vi "LogonUser.vi"() -> ()   [LabVIEW 2018]
doc: "©2019\nWiebe Walstra\nwww.carya.nl"
uses:
  kernel32.dll
  advapi32.dll
panel:
  out "Name before":string
  out "success 4":i32
  out "success 3":i32
  out "success 2":i32
  out "error out":errorcluster
  out "Name during":string
  out "Name after":string
  out "error":i32
  out "success":i32
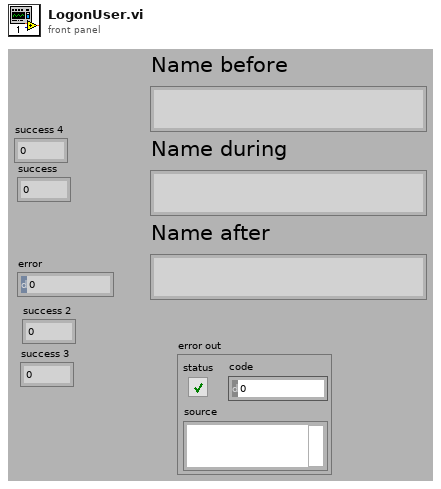
[diagram p1: front panel]
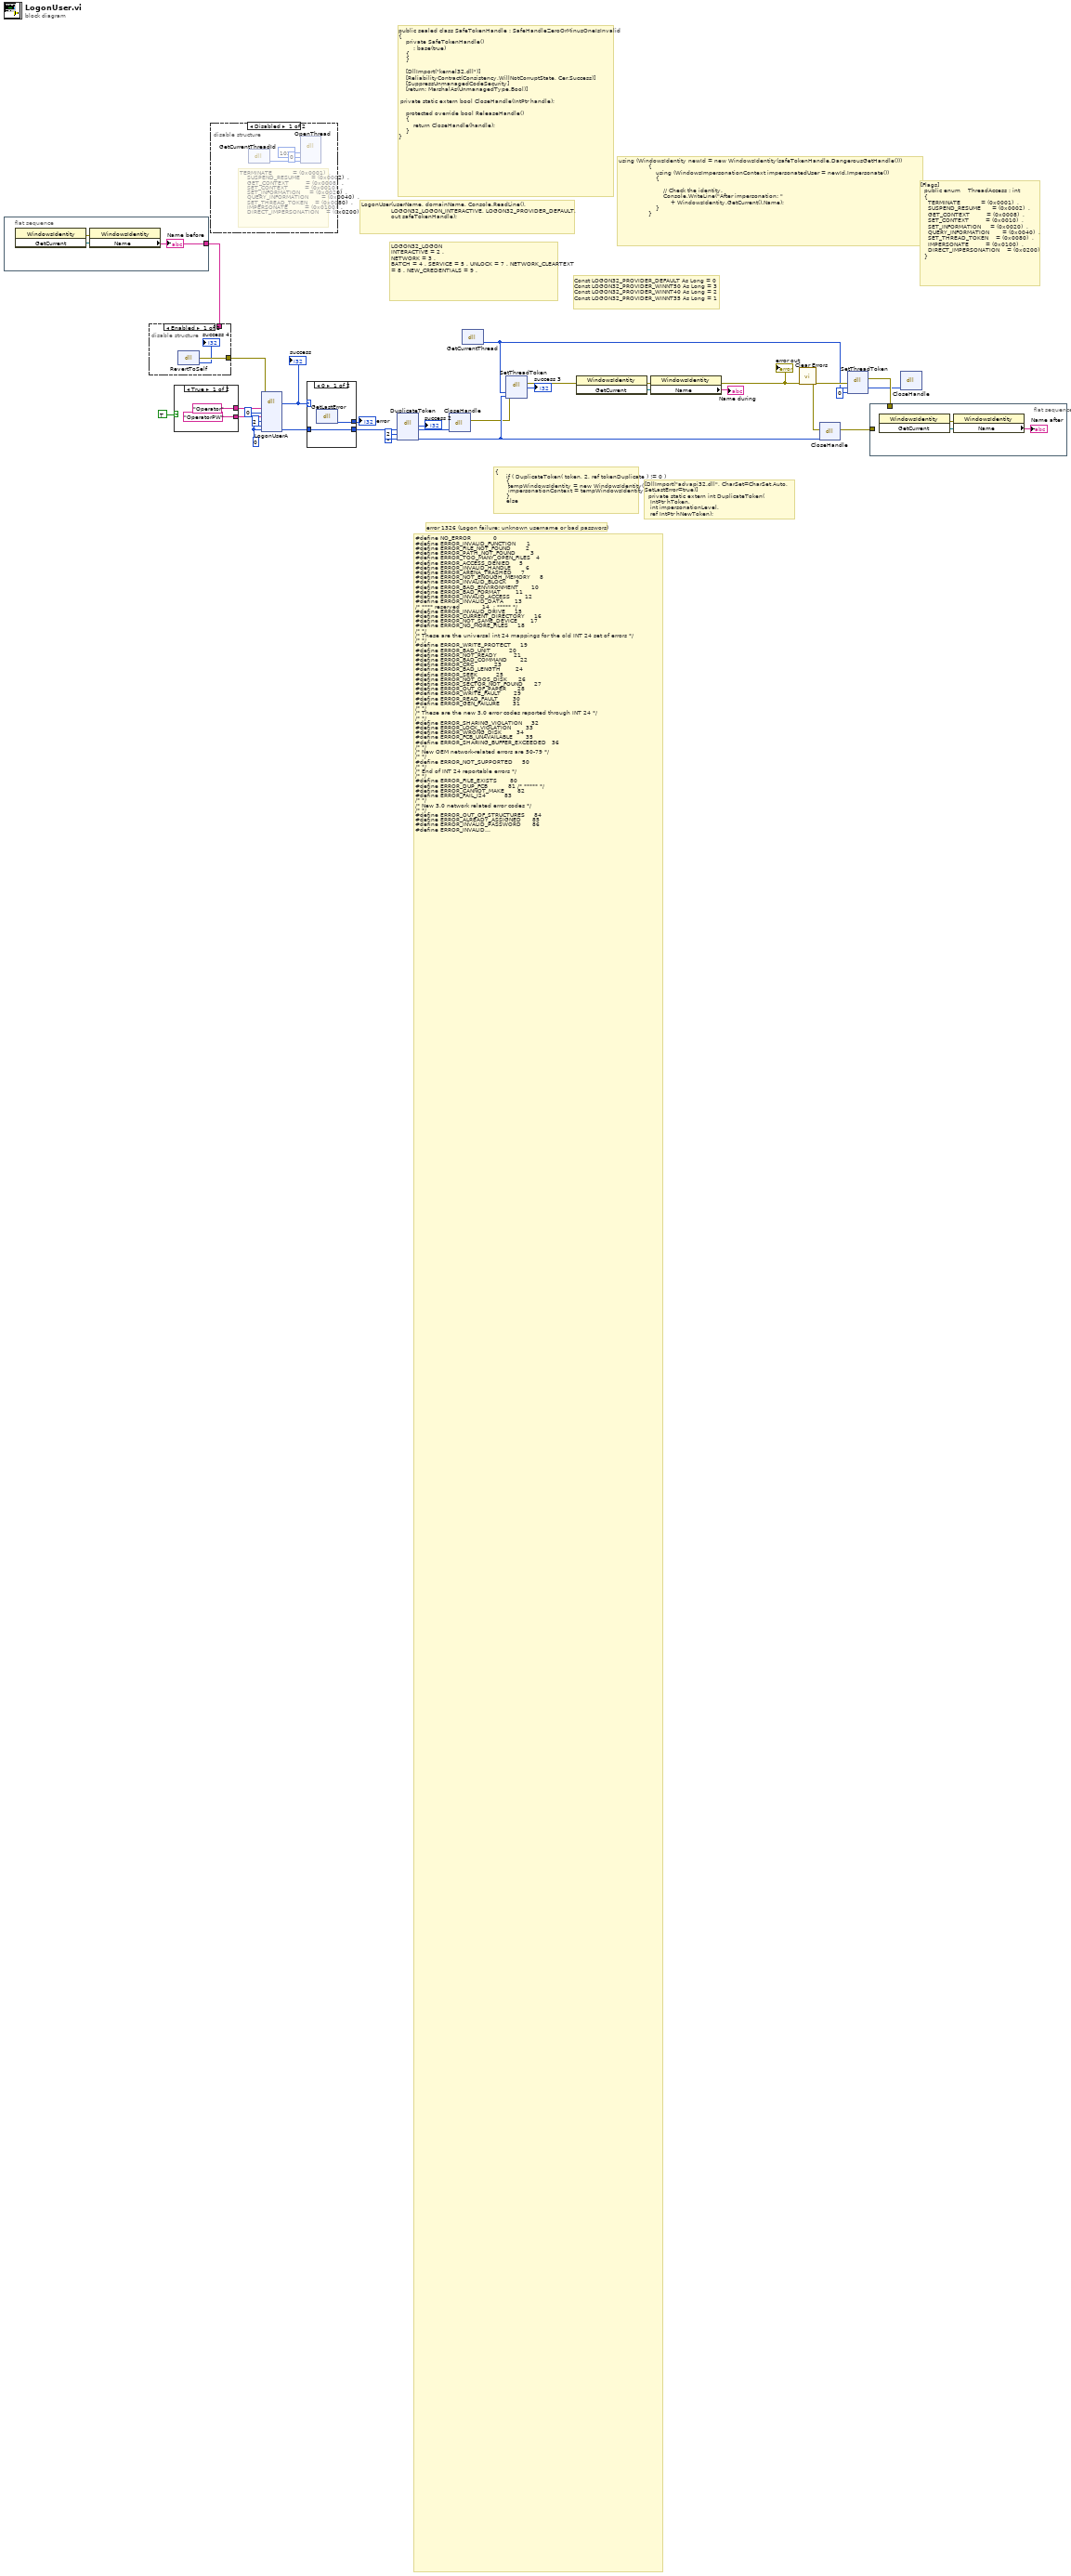
[diagram p0: block diagram]
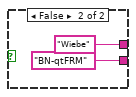
[diagram p5: hidden frame]
diagram:
  w27 = 0 ("dwLogonType")
  # "[Flags]\n  public enum    ThreadAccess : int\n  {\n    TERMINATE           = (0x0001)  ,\n    SUSPEND_RESUME      = (0x0002)  ,\n    GET_CONTEXT         = (0x0008)  ,\n    SET_CONTEXT         = (0x0010)  ,\n    SET_INFORMATION     = (0x0020)  ,\n    QUERY_INFORMATION       = (0x0040)  ,\n    SET_THREAD_TOKEN    = (0x0080)  ,\n    IMPERSONATE         = (0x0100)  ,\n    DIRECT_IMPERSONATION    = (0x0200)\n  }"
  # "[DllImport(\"advapi32.dll\", CharSet=CharSet.Auto, SetLastError=true)]\n\t\tprivate static extern int DuplicateToken(\n\t\t\tIntPtr hToken,\n\t\t\tint impersonationLevel,\n\t\t\tref IntPtr hNewToken);"
  # "{\n\t\t\t\t\t\tif ( DuplicateToken( token, 2, ref tokenDuplicate ) != 0 )\n\t\t\t\t\t\t{\n\t\t\t\t\t\t\ttempWindowsIdentity = new WindowsIdentity( tokenDuplicate );\n\t\t\t\t\t\t\timpersonationContext = tempWindowsIdentity.Impersonate();\n\t\t\t\t\t\t}\n\t\t\t\t\t\telse"
  # "public sealed class SafeTokenHandle : SafeHandleZeroOrMinusOneIsInvalid\n{\n    private SafeTokenHandle()\n        : base(true)\n    {\n    }\n\n    [DllImport(\"kernel32.dll\")]\n    [ReliabilityContract(Consistency.WillNotCorruptState, Cer.Success)]\n    [SuppressUnmanagedCodeSecurity]\n    [return: MarshalAs(UnmanagedType.Bool)]\n  \n private static extern bool CloseHandle(IntPtr handle);\n\n    protected override bool ReleaseHandle()\n    {\n        return CloseHandle(handle);\n    }\n}"
  # "LogonUser(userName, domainName, Console.ReadLine(),\n                LOGON32_LOGON_INTERACTIVE, LOGON32_PROVIDER_DEFAULT,\n                out safeTokenHandle);"
  # "using (WindowsIdentity newId = new WindowsIdentity(safeTokenHandle.DangerousGetHandle()))\n                {\n                    using (WindowsImpersonationContext impersonatedUser = newId.Impersonate())\n                    {\n\n                        // Check the identity.\n                        Console.WriteLine(\"After impersonation: \"\n                            + WindowsIdentity.GetCurrent().Name);\n                    }\n                }"
  # "Const LOGON32_PROVIDER_DEFAULT As Long = 0\nConst LOGON32_PROVIDER_WINNT50 As Long = 3\nConst LOGON32_PROVIDER_WINNT40 As Long = 2\nConst LOGON32_PROVIDER_WINNT35 As Long = 1"
  # "error 1326 (Logon failure: unknown username or bad passwors)"
  # "LOGON32_LOGON \nINTERACTIVE = 2 .\nNETWORK = 3 .\nBATCH = 4 . SERVICE = 5 . UNLOCK = 7 . NETWORK_CLEARTEXT = 8 . NEW_CREDENTIALS = 9 ."
  # "#define NO_ERROR            0\n#define ERROR_INVALID_FUNCTION      1\n#define ERROR_FILE_NOT_FOUND        2\n#define ERROR_PATH_NOT_FOUND        3\n#define ERROR_TOO_MANY_OPEN_FILES   4\n#define ERROR_ACCESS_DENIED     5\n#define ERROR_INVALID_HANDLE        6\n#define ERROR_ARENA_TRASHED     7\n#define ERROR_NOT_ENOUGH_MEMORY     8\n#define ERROR_INVALID_BLOCK     9\n#define ERROR_BAD_ENVIRONMENT       10\n#define ERROR_BAD_FORMAT        11\n#define ERROR_INVALID_ACCESS        12\n#define ERROR_INVALID_DATA      13\n/* **** reserved            14  ; ***** */\n#define ERROR_INVALID_DRIVE     15\n#define ERROR_CURRENT_DIRECTORY     16\n#define ERROR_NOT_SAME_DEVICE       17\n#define ERROR_NO_MORE_FILES     18\n/* */\n/* These are the universal int 24 mappings for the old INT 24 set of errors */\n/* */\n#define ERROR_WRITE_PROTECT     19\n#define ERROR_BAD_UNIT          20\n#define ERROR_NOT_READY         21\n#define ERROR_BAD_COMMAND       22\n#define ERROR_CRC           23\n#define ERROR_BAD_LENGTH        24\n#define ERROR_SEEK          25\n#define ERROR_NOT_DOS_DISK      26\n#define ERROR_SECTOR_NOT_FOUND      27\n#define ERROR_OUT_OF_PAPER      28\n#define ERROR_WRITE_FAULT       29\n#define ERROR_READ_FAULT        30\n#define ERROR_GEN_FAILURE       31\n/* */\n/* These are the new 3.0 error codes reported through INT 24 */\n/* */\n#define ERROR_SHARING_VIOLATION     32\n#define ERROR_LOCK_VIOLATION        33\n#define ERROR_WRONG_DISK        34\n#define ERROR_FCB_UNAVAILABLE       35\n#define ERROR_SHARING_BUFFER_EXCEEDED   36\n/* */\n/* New OEM network-related errors are 50-79 */\n/* */\n#define ERROR_NOT_SUPPORTED     50\n/* */\n/* End of INT 24 reportable errors */\n/* */\n#define ERROR_FILE_EXISTS       80\n#define ERROR_DUP_FCB           81 /* ***** */\n#define ERROR_CANNOT_MAKE       82\n#define ERROR_FAIL_I24          83\n/* */\n/* New 3.0 network related error codes */\n/* */\n#define ERROR_OUT_OF_STRUCTURES     84\n#define ERROR_ALREADY_ASSIGNED      85\n#define ERROR_INVALID_PASSWORD      86\n#define ERROR_INVALID_PARAMETER     87\n#define ERROR_NET_WRITE_FAULT       88\n/* */\n/* New error codes for 4.0 */\n/* */\n#define ERROR_NO_PROC_SLOTS     89  /* no process slots available */\n#define ERROR_NOT_FROZEN        90\n#define ERR_TSTOVFL         91  /* timer service table overflow */\n#define ERR_TSTDUP          92  /* timer service table duplicate */\n#define ERROR_NO_ITEMS          93  /* There were no items to operate upon */\n#define ERROR_INTERRUPT         95  /* interrupted system call */\n\n#define ERROR_TOO_MANY_SEMAPHORES   100\n#define ERROR_EXCL_SEM_ALREADY_OWNED    101\n#define ERROR_SEM_IS_SET        102\n#define ERROR_TOO_MANY_SEM_REQUESTS 103\n#define ERROR_INVALID_AT_INTERRUPT_TIME 104\n\n#define ERROR_SEM_OWNER_DIED        105 /* waitsem found owner died */\n#define ERROR_SEM_USER_LIMIT        106 /* too many procs have this sem */\n#define ERROR_DISK_CHANGE       107 /* insert disk b into drive a */\n#define ERROR_DRIVE_LOCKED      108 /* drive locked by another process */\n#define ERROR_BROKEN_PIPE       109 /* write on pipe with no reader */\n/* */\n/* New error codes for OS/2 */\n/* */\n#define ERROR_OPEN_FAILED       110 /* open/created failed due to */\n                        /* explicit fail command */\n#define ERROR_BUFFER_OVERFLOW       111 /* buffer passed to system call */\n                        /* is too small to hold return */\n                        /* data. */\n#define ERROR_DISK_FULL         112 /* not enough space on the disk */\n                        /* (DOSNEWSIZE/w_NewSize) */\n#define ERROR_NO_MORE_SEARCH_HANDLES    113 /* can't allocate another search */\n                        /* structure and handle. */\n                        /* (DOSFINDFIRST/w_FindFirst) */\n#define ERROR_INVALID_TARGET_HANDLE 114 /* Target handle in DOSDUPHANDLE */\n                        /* is invalid */\n#define ERROR_PROTECTION_VIOLATION  115 /* Bad user virtual address */\n#define ERROR_VIOKBD_REQUEST        116\n#define ERROR_INVALID_CATEGORY      117 /* Category for DEVIOCTL in not */\n                        /* defined */\n#define ERROR_INVALID_VERIFY_SWITCH 118 /* invalid value passed for */\n                        /* verify flag */\n#define ERROR_BAD_DRIVER_LEVEL      119 /* DosDevIOCTL looks for a level */\n                        /* four driver.   If the driver */\n                        /* is not level four we return */\n                        /* this code */\n#define ERROR_CALL_NOT_IMPLEMENTED  120 /* returned from stub api calls. */\n                        /* This call will disappear when */\n                        /* all the api's are implemented. */\n#define ERROR_SEM_TIMEOUT       121 /* Time out happened from the */\n                        /* semaphore api functions. */\n#define ERROR_INSUFFICIENT_BUFFER   122 /* Some call require the  */\n                        /* application to pass in a buffer */\n                        /* filled with data.  This error is */\n                        /* returned if the data buffer is too */\n                        /* small.  For example: DosSetFileInfo */\n                        /* requires 4 bytes of data.  If a */\n                        /* two byte buffer is passed in then */\n                        /* this error is returned.   */\n                        /* error_buffer_overflow is used when */\n                        /* the output buffer in not big enough. */\n#define ERROR_INVALID_NAME      123 /* illegal character or malformed */\n                        /* file system name */\n#define ERROR_INVALID_LEVEL     124 /* unimplemented level for info */\n                        /* retrieval or setting */\n#define ERROR_NO_VOLUME_LABEL       125 /* no volume label found with */\n                        /* DosQFSInfo command */\n#define ERROR_MOD_NOT_FOUND     126 /* w_getprocaddr,w_getmodhandle */\n#define ERROR_PROC_NOT_FOUND        127 /* w_getprocaddr */\n\n#define ERROR_WAIT_NO_CHILDREN      128 /* CWait finds to children */\n\n#define ERROR_CHILD_NOT_COMPLETE    129 /* CWait children not dead yet */\n\n/*This is a temporary fix for the 4-19-86 build this should be changed when */\n/* we get the file from MS */\n#define ERROR_DIRECT_ACCESS_HANDLE  130 /* handle operation is invalid */\n                        /* for direct disk access */\n                        /* handles */\n#define ERROR_NEGATIVE_SEEK     131 /* application tried to seek  */\n                        /* with negative offset */\n#define ERROR_SEEK_ON_DEVICE        132 /* application tried to seek */\n                        /* on device or pipe */\n/* */\n/* The following are errors generated by the join and subst workers */\n/* */\n#define ERROR_IS_JOIN_TARGET        133\n#define ERROR_IS_JOINED         134\n#define ERROR_IS_SUBSTED        135\n#define ERROR_NOT_JOINED        136\n#define ERROR_NOT_SUBSTED       137\n#define ERROR_JOIN_TO_JOIN      138\n#define ERROR_SUBST_TO_SUBST        139\n#define ERROR_JOIN_TO_SUBST     140\n#define ERROR_SUBST_TO_JOIN     141\n#define ERROR_BUSY_DRIVE        142\n#define ERROR_SAME_DRIVE        143\n#define ERROR_DIR_NOT_ROOT      144\n#define ERROR_DIR_NOT_EMPTY     145\n#define ERROR_IS_SUBST_PATH     146\n#define ERROR_IS_JOIN_PATH      147\n#define ERROR_PATH_BUSY         148\n#define ERROR_IS_SUBST_TARGET       149\n#define ERROR_SYSTEM_TRACE      150 /* system trace error */\n#define ERROR_INVALID_EVENT_COUNT   151 /* DosMuxSemWait errors */\n#define ERROR_TOO_MANY_MUXWAITERS   152\n#define ERROR_INVALID_LIST_FORMAT   153\n#define ERROR_LABEL_TOO_LONG        154\n#define ERROR_TOO_MANY_TCBS     155\n#define ERROR_SIGNAL_REFUSED        156\n#define ERROR_DISCARDED         157\n#define ERROR_NOT_LOCKED        158\n#define ERROR_BAD_THREADID_ADDR     159\n#define ERROR_BAD_ARGUMENTS     160\n#define ERROR_BAD_PATHNAME      161\n#define ERROR_SIGNAL_PENDING        162\n#define ERROR_UNCERTAIN_MEDIA       163\n#define ERROR_MAX_THRDS_REACHED     164\n#define ERROR_MONITORS_NOT_SUPPORTED    165\n\n#define ERROR_INVALID_SEGMENT_NUMBER    180\n#define ERROR_INVALID_CALLGATE      181\n#define ERROR_INVALID_ORDINAL       182\n#define ERROR_ALREADY_EXISTS        183\n#define ERROR_NO_CHILD_PROCESS      184\n#define ERROR_CHILD_ALIVE_NOWAIT    185\n#define ERROR_INVALID_FLAG_NUMBER   186\n#define ERROR_SEM_NOT_FOUND     187\n\n/*  following error codes have added to make the loader error\n    messages distinct\n*/\n\n#define ERROR_INVALID_STARTING_CODESEG  188\n#define ERROR_INVALID_STACKSEG      189\n#define ERROR_INVALID_MODULETYPE    190\n#define ERROR_INVALID_EXE_SIGNATURE 191\n#define ERROR_EXE_MARKED_INVALID    192\n#define ERROR_BAD_EXE_FORMAT        193\n#define ERROR_ITERATED_DATA_EXCEEDS_64k 194\n#define ERROR_INVALID_MINALLOCSIZE  195\n#define ERROR_DYNLINK_FROM_INVALID_RING 196\n#define ERROR_IOPL_NOT_ENABLED      197\n#define ERROR_INVALID_SEGDPL        198\n#define ERROR_AUTODATASEG_EXCEEDS_64k   199\n#define ERROR_RING2SEG_MUST_BE_MOVABLE  200\n#define ERROR_RELOC_CHAIN_XEEDS_SEGLIM  201\n#define ERROR_INFLOOP_IN_RELOC_CHAIN    202\n\n#define ERROR_ENVVAR_NOT_FOUND      203\n#define ERROR_NOT_CURRENT_CTRY      204\n#define ERROR_NO_SIGNAL_SENT        205\n#define ERROR_FILENAME_EXCED_RANGE  206 /* if filename > 8.3 */\n#define ERROR_RING2_STACK_IN_USE    207 /* for FAPI */\n#define ERROR_META_EXPANSION_TOO_LONG   208 /* if \"*a\" > 8.3 */\n\n#define ERROR_INVALID_SIGNAL_NUMBER 209\n#define ERROR_THREAD_1_INACTIVE     210\n#define ERROR_INFO_NOT_AVAIL        211 /*@@ PTM 5550 */\n#define ERROR_LOCKED            212\n#define ERROR_BAD_DYNALINK      213 /*@@ PTM 5760 */\n#define ERROR_TOO_MANY_MODULES      214\n#define ERROR_NESTING_NOT_ALLOWED   215\n\n/*\n * Error codes 230 - 249 are reserved for MS Networks\n */\n\n#define ERROR_USER_DEFINED_BASE     0xF000\n\n#define ERROR_I24_WRITE_PROTECT     0\n#define ERROR_I24_BAD_UNIT      1\n#define ERROR_I24_NOT_READY     2\n#define ERROR_I24_BAD_COMMAND       3\n#define ERROR_I24_CRC           4\n#define ERROR_I24_BAD_LENGTH        5\n#define ERROR_I24_SEEK          6\n#define ERROR_I24_NOT_DOS_DISK      7\n#define ERROR_I24_SECTOR_NOT_FOUND  8\n#define ERROR_I24_OUT_OF_PAPER      9\n#define ERROR_I24_WRITE_FAULT       0x0A\n#define ERROR_I24_READ_FAULT        0x0B\n#define ERROR_I24_GEN_FAILURE       0x0C\n#define ERROR_I24_DISK_CHANGE       0x0D\n#define ERROR_I24_WRONG_DISK        0x0F\n#define ERROR_I24_UNCERTAIN_MEDIA   0x10\n#define ERROR_I24_CHAR_CALL_INTERRUPTED 0x11\n#define ERROR_I24_NO_MONITOR_SUPPORT    0x12\n#define ERROR_I24_INVALID_PARAMETER 0x13"
  n1 = flat-sequence {
    tunnel: [w31] -> w13
    frame #0 {
      n2 = invoke class="WindowsIdentity" method="GetCurrent"() -> (error out=w32:errorcluster, "GetCurrent"=w33:refnum<k24>)  [unwired: 3 in, 1 out]
      n3 = property class="WindowsIdentity"(reference=w33, error in=w32) -> ("Name"=w31:string)  [unwired: 2 out]
      "Name before" <- w31
    }
  }
  n4 = disable-structure shown="Enabled" {
    disable-tunnel: [w35 _] -> w18
    disable-tunnel: w13 -> [_ _]
    frame Enabled {
      n5 = dll-call lib="Advapi32.dll" fn="RevertToSelf"() -> (error out=w35:errorcluster, "success"=→"success 4":i32)  [unwired: 3 in, 1 out]
    }
    frame Disabled {
    }
  }
  n6 = case shown="True" TRUE ("Case Constant\n(See Context Help)") {
    tunnel: ["Operator" ("username") "Wiebe" ("username")] -> w11
    tunnel: ["OperatorPW" ("password") "BN-qtFRM" ("password")] -> w30
    frame True {
    }
    frame False {
    }
  }
  n7 = disable-structure shown="Disabled" {
    frame Disabled {
      # "TERMINATE           = (0x0001)  ,\n    SUSPEND_RESUME      = (0x0002)  ,\n    GET_CONTEXT         = (0x0008)  ,\n    SET_CONTEXT         = (0x0010)  ,\n    SET_INFORMATION     = (0x0020)  ,\n    QUERY_INFORMATION       = (0x0040)  ,\n    SET_THREAD_TOKEN    = (0x0080)  ,\n    IMPERSONATE         = (0x0100)  ,\n    DIRECT_IMPERSONATION    = (0x0200)"
      n8 = dll-call lib="kernel32.dll" fn="GetCurrentThreadId"() -> ("thread"=w40:i64)  [unwired: 3 in, 2 out]
      n9 = dll-call lib="kernel32.dll" fn="OpenThread"("dwDesiredAccess"=1023 ("bInheritHandle"), "bInheritHandle"=0, "ThreadID"=w40) -> ()  [unwired: 7 in, 2 out]
    }
    frame Enabled {
    }
  }
  n10 = dll-call lib="Advapi32.dll" fn="LogonUserA"(error in=w18, "username"=w11, "domain"=0, "password"=w30, "dwLogonType"=2, "dwLogonProvider"=w27, "phToken"=w27) -> ("success"=w25:i32, "phToken"=w28:i64)  [unwired: 7 in, 2 out]
  "success" <- w25
  n11 = case shown="0" w25 {
    tunnel: w28 -> [w44 w45]
    tunnel: [w44 w45] -> w5
    tunnel: [w43 _] -> w23
    frame 0 {
      n12 = dll-call lib="kernel32.dll" fn="GetLastError"() -> ("error"=w43:i32)  [unwired: 3 in, 2 out]
    }
    frame Default {
    }
  }
  "error" <- w23
  n13 = dll-call lib="Advapi32.dll" fn="DuplicateToken"("phToken"=w5, "impersonationLevel"=2, "newToken"=i64 0) -> ("success"=→"success 2":i32, "phToken"=w6:i64, "newToken"=w14:i64)  [unwired: 4 in, 2 out]
  n14 = dll-call lib="kernel32.dll" fn="CloseHandle"("handle"=w6) -> (error out=w4:errorcluster)  [unwired: 5 in, 1 out]
  n15 = dll-call lib="kernel32.dll" fn="GetCurrentThread"() -> ("thread"=w3:i64)  [unwired: 3 in, 2 out]
  n16 = dll-call lib="Advapi32.dll" fn="SetThreadToken"(error in=w4, "pThread"=w3, "newToken"=w14) -> (error out=w12:errorcluster, "success"=→"success 3":i32)  [unwired: 4 in, 1 out]
  n17 = invoke class="WindowsIdentity" method="GetCurrent"(error in=w12) -> (error out=w10:errorcluster, "GetCurrent"=w9:refnum<k24>)  [unwired: 2 in, 1 out]
  n18 = property class="WindowsIdentity"(reference=w9, error in=w10) -> (error out=w21:errorcluster, "Name"=→"Name during":string)  [unwired: 1 out]
  "error out" <- w21
  n19 = call <vilib>:"Clear Errors.vi"("error in (no error)"=w21) -> ("error out"=w7:errorcluster)  [unwired: 5 in, 1 out]
  n20 = dll-call lib="kernel32.dll" fn="CloseHandle"(error in=w7, "handle"=w14) -> (error out=w22:errorcluster)  [unwired: 4 in, 1 out]
  n21 = dll-call lib="Advapi32.dll" fn="SetThreadToken"(error in=w7, "pThread"=w3, "newToken"=i64 0) -> (error out=w16:errorcluster, "pThread"=w1:i64)  [unwired: 4 in, 1 out]
  n22 = flat-sequence {
    tunnel: w22 -> [_]
    tunnel: w16 -> [_]
    frame #0 {
      n23 = invoke class="WindowsIdentity" method="GetCurrent"() -> (error out=w46:errorcluster, "GetCurrent"=w47:refnum<k24>)  [unwired: 3 in, 1 out]
      n24 = property class="WindowsIdentity"(reference=w47, error in=w46) -> ("Name"=→"Name after":string)  [unwired: 2 out]
    }
  }
  n25 = dll-call lib="kernel32.dll" fn="CloseHandle"("handle"=w1) -> ()  [unwired: 5 in, 2 out]
